vi "Frame create.vi"(7 "Command":string, 8 "error in (no error)":errorcluster, 11 "ISO 14443 B UP in":refnum<class "ISO 14443 B UP.lvclass">) -> (0 "error out":errorcluster, 3 "ISO 14443 B UP out":refnum<class "ISO 14443 B UP.lvclass">)   [LabVIEW 2019, in "ISO 14443 B UP.lvclass"]
uses:
  ISO 14443 B UP.lvclass
  TypeDef/Store.ctl
  ISO 14443 B UP.lvclass/ISO 14443 B UP.ctl
  RFID system.lvclass
panel:
  in  "PUPI":u8[](array[numeric])=[178, 212, 178, 212] format="%x"
  in  "1":u8[](array[numeric])=[80] format="%x"
  in  "App data":u8[](array[numeric])=[213, 18, 68, 243] format="%x"
  in  "Protocol Info":u8[](array[numeric])=[3, 18, 227] format="%x"
  # "App data"
  # "Protocol info"
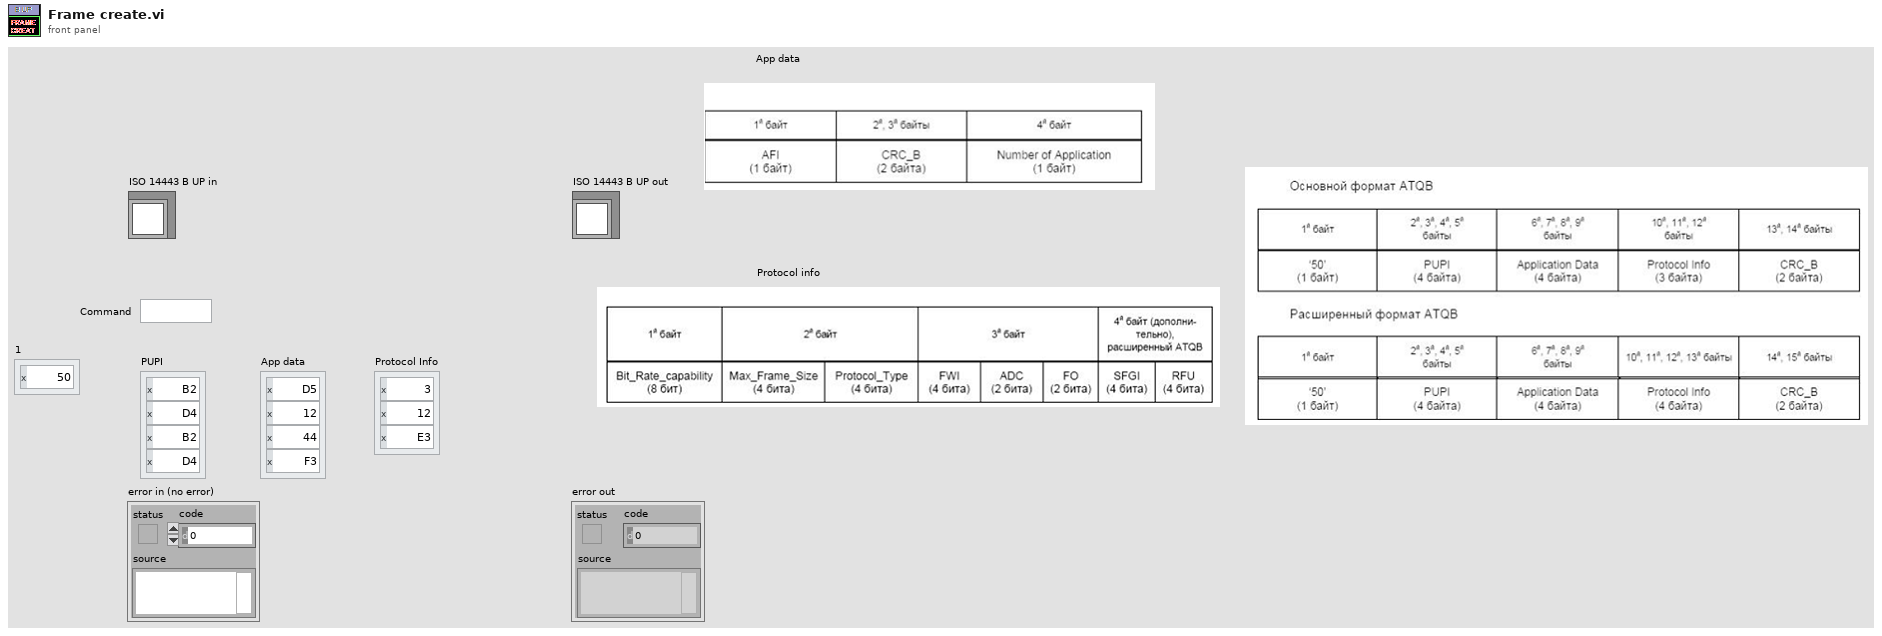
[diagram p1: front panel]
types:
  T1 = typedef "Store.ctl" = enum16{"envelope", "noise", "demSubCar", "CH_frame", "Decode", "demodulate", "in", "out", "sum", "subCarrier", "frame", "command", "encode", "modulate", "encode_UP", "modulate_up", "demod_up", "envelop_up", "sum_up", "out_up", "in_up"}
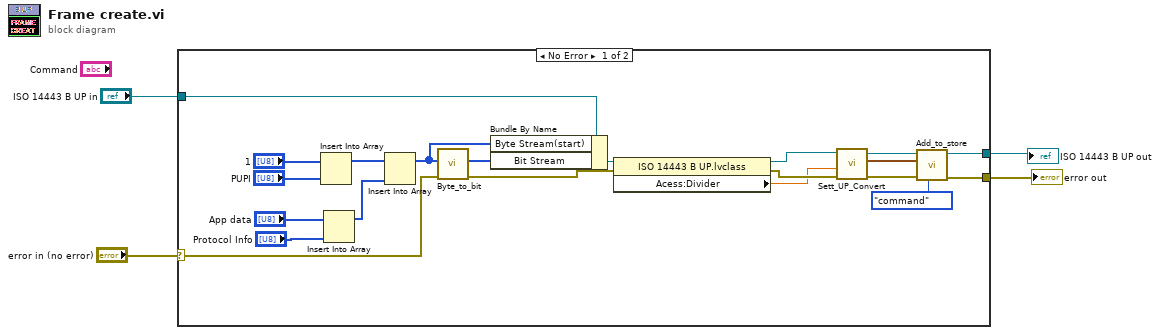
[diagram p0: block diagram]
diagram:
  n1 = case shown="No Error" "error in (no error)" {
    selector: "error in (no error)" -> [w19 w26]
    tunnel: [w11 w26] -> w1
    tunnel: "ISO 14443 B UP in" -> [w18 w27]
    tunnel: [w14 w27] -> w2
    frame No Error {
      n2 = Insert Into Array(array="1", new element="PUPI") -> (w23:u8[])  [unwired: 1 in]
      n3 = Insert Into Array(array="App data", new element="Protocol Info") -> (w20:u8[])  [unwired: 1 in]
      n4 = Insert Into Array(array=w23, new element=w20) -> (w5:u8[])  [unwired: 1 in]
      n5 = call "Byte_to_bit.vi"("Error In"=w19, "Array of byte"=w5) -> ("Error Out"=w8:errorcluster, "Arrray of bit"=w17:u8[])  [unwired: 5 in, 1 out]
      n6 = Bundle By Name(cluster=w18, "Byte Stream(start)"=w5, "Bit Stream"=w17) -> (w16:refnum<class "ISO 14443 B UP.lvclass">)
      n7 = property class="ISO 14443 B UP.lvclass"(reference=w16, error in=w8) -> (reference out=w9:refnum<class "ISO 14443 B UP.lvclass">, error out=w7:errorcluster, "Acess:Divider"=w6:dbl)
      n8 = call-dynamic "Sett_UP_Convert.vi"("error in (no error)"=w7, "Divider(1)"=w6, "ISO 14443 B UP in"=w9) -> ("error out"=w13:errorcluster, "Waveform"=w12:waveform(dbl), "ISO 14443 B UP out"=w15:refnum<class "ISO 14443 B UP.lvclass">)  [unwired: 6 in]
      n9 = call "Add_to_store.vi"("Store"=Store."command", "error in (no error)"=w13, "Waveform"=w12, "RFID system in"=w15) -> ("error out"=w11:errorcluster, "RFID system out"=w14:refnum<class "ISO 14443 B UP.lvclass">)  [unwired: 6 in]
    }
    frame Error {
    }
  }
  "error out" <- w1
  "ISO 14443 B UP out" <- w2
